vi "dyanic event adavnce.vi"() -> ()   [LabVIEW 2022 SP3]
panel:
  in  "stop 2":bool
  in  "stop":bool
  out "Message":string
  out "Bool":bool
  out "Numeric":dbl
  in  "String":string
  in  "Boolean":bool
  in  "Thermometer":dbl(slide) scale=0.0..100.0
  # "Publisher"
  # "Subscriber"
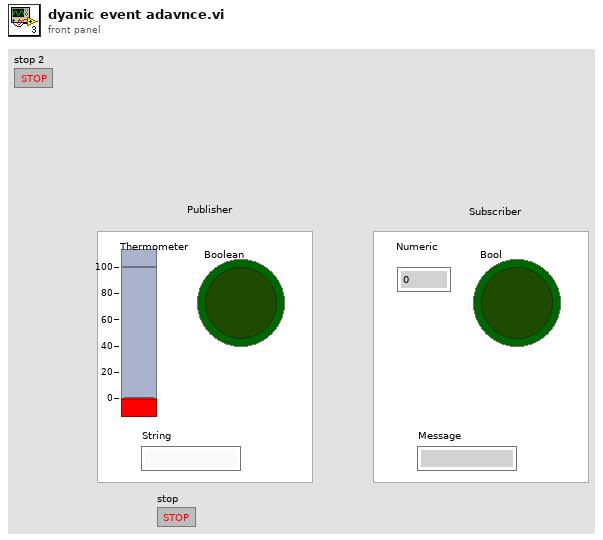
[diagram p1: front panel]
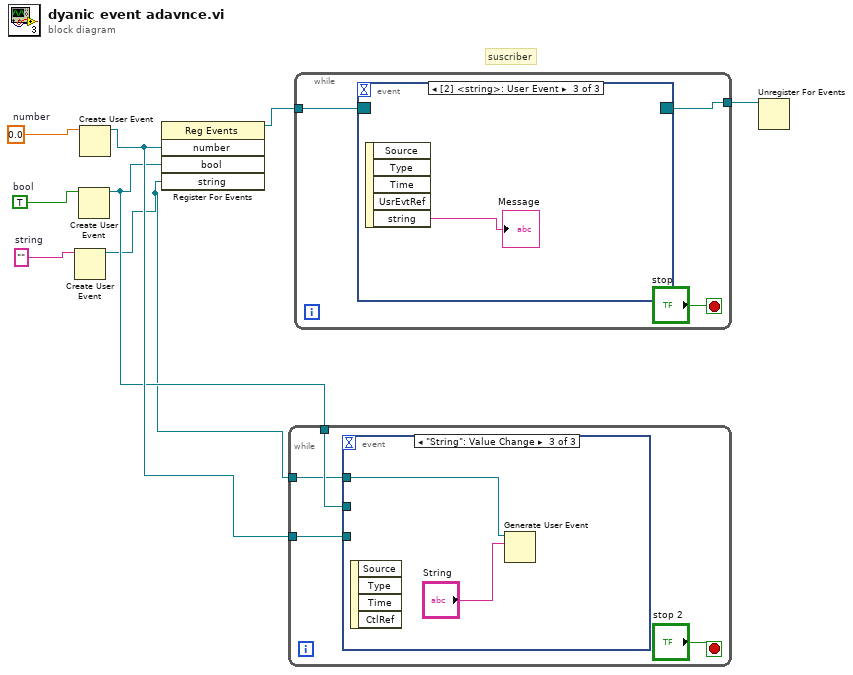
[diagram p0: block diagram]
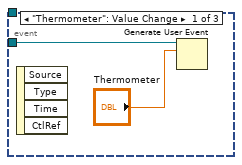
[diagram p2: hidden frame]
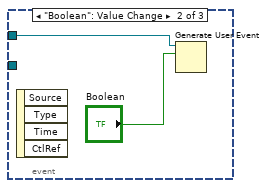
[diagram p3: hidden frame]
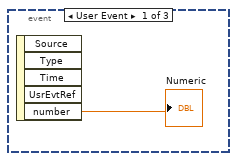
[diagram p4: hidden frame]
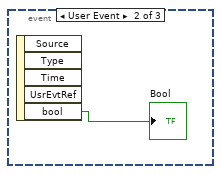
[diagram p5: hidden frame]
diagram:
  w6 = ""  # string
  w7 = TRUE  # bool
  w8 = 0.0  # number
  # "suscriber"
  n1 = Create User Event(user event datatype=w6) -> (user event=w1:refnum<user-event>)  [unwired: 1 in, 1 out]
  n2 = Create User Event(user event datatype=w7) -> (user event=w2:refnum<user-event>)  [unwired: 1 in, 1 out]
  n3 = Create User Event(user event datatype=w8) -> (user event=w3:refnum<user-event>)  [unwired: 1 in, 1 out]
  n4 = register-events(w3, w2, w1) -> (reference out=w5:refnum<event-registration>)  [unwired: 2 in, 1 out]
  n5 = while {
    tunnel: w3 -> [w11]
    tunnel: w2 -> [w10]
    tunnel: w1 -> [w9]
    stop <- "stop 2" stop-if-true
    n6 = event shown="[2] \"String\": Value Change" {
      selector: _ -> [_ _ _]
      dyn-events: _ -> [_ _ _]
      timeout: _ -> [_ _ _]
      tunnel: w11 -> [w13 _ _]
      tunnel: w10 -> [_ w15 _]
      tunnel: w9 -> [_ _ w18]
      event "Thermometer": Value Change {
        n7 = event-data() -> ()  [unwired: 1 in, 4 out]
        n8 = Generate User Event(user event=w13, event data cluster="Thermometer") -> ()  [unwired: 2 in, 2 out]
      }
      event "Boolean": Value Change {
        n9 = event-data() -> ()  [unwired: 1 in, 4 out]
        n10 = Generate User Event(user event=w15, event data cluster="Boolean") -> ()  [unwired: 2 in, 2 out]
      }
      event "String": Value Change {
        n11 = event-data() -> ()  [unwired: 1 in, 4 out]
        n12 = Generate User Event(user event=w18, event data cluster="String") -> ()  [unwired: 2 in, 2 out]
      }
    }
  }
  n13 = while {
    tunnel: w5 -> [w20]
    tunnel: [w19] -> w4
    stop <- "stop" stop-if-true
    n14 = event shown="[2] <string>: User Event" {
      selector: w20 -> [_ _ _]
      dyn-events: [_ _ _] -> w19
      timeout: _ -> [_ _ _]
      event User Event {
        n15 = event-data() -> ("number"=→"Numeric":dbl)  [unwired: 1 in, 4 out]
      }
      event User Event {
        n16 = event-data() -> ("bool"=→"Bool":bool)  [unwired: 1 in, 4 out]
      }
      event User Event {
        n17 = event-data() -> ("string"=→"Message":string)  [unwired: 1 in, 4 out]
      }
    }
  }
  n18 = Unregister For Events(event registration refnum=w4) -> ()  [unwired: 1 in, 1 out]
